vi "SerialReadLine.vi"(8 "error in":errorcluster, 11 "VISA resource name in":refnum<visa-resource-name>) -> (0 "error out":errorcluster, 2 "String":string, 3 "VISA resource name out":refnum<visa-resource-name>)   [LabVIEW 2017]
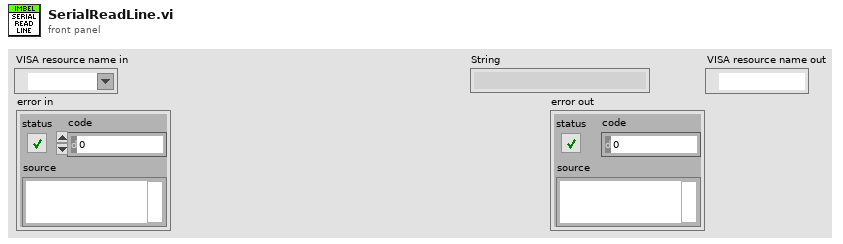
[diagram p1: front panel]
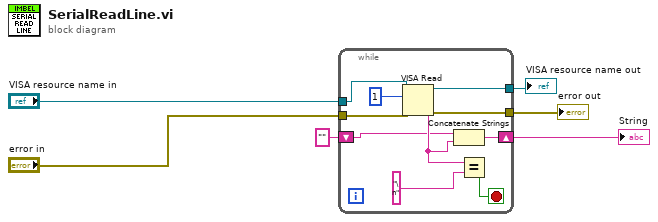
[diagram p0: block diagram]
diagram:
  n1 = while {
    tunnel: "error in" -> [w15]
    tunnel: [w13] -> w4
    tunnel: [w12] -> w5
    shift-right: [w10] -> w6
    shift-left: "" -> [w8]
    tunnel: "VISA resource name in" -> [w7]
    stop <- w11 stop-if-true
    n2 = VISA Read(VISA resource name=w7, byte count=u32 1, error in (no error)=w15) -> (VISA resource name out=w13:refnum<visa-resource-name>, read buffer=w9:string, error out=w12:errorcluster)  [unwired: 1 out]
    n3 = Concatenate Strings(w8, w9) -> (w10:string)
    n4 = Equal?(x=w9, y="\n" ("String 2")) -> (x = y?=w11:bool)
  }
  "String" <- w6
  "error out" <- w5
  "VISA resource name out" <- w4
